vi "TraverseControl_High.vi"(0 "Mode":T1=enum."Read traverse position", 1 "Route Checking?":bool, 3 "Traverse Name":string, 7 "Model       Roll      Pitch       Yaw (deg)":dbl[](array[numeric]) format="%#.2f", 11 "Position input XYZ":dbl[](array[numeric])=[0.0, 0.0, 0.0] format="%.2f", 13 "Speed Factor":dbl=1.0 min=0.1 max=5.0 format="%.2f", 14 "Backlash Compensation?":bool=TRUE) -> (4 "Position Output XYZ":dbl[](array[numeric]) format="%.2f", 15 "Error String":string)   [LabVIEW 2012]
uses:
  Anemometry/Anemometry Sub Vis/Gen Trav/Trav_mode.ctl
  Anemometry/Anemometry Sub Vis/Globals/Trav_pos_global.vi
  Anemometry/Anemometry Sub Vis/Gen Trav/Route mapping/Route_mapping_global.vi
  Anemometry/Anemometry Sub Vis/Globals/Preference_global.vi
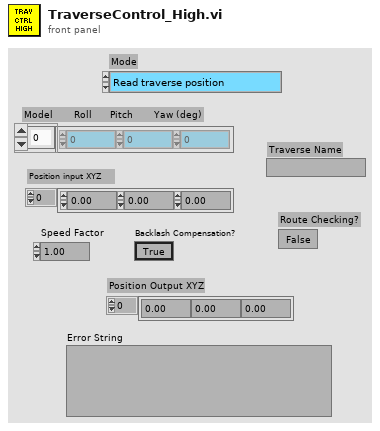
[diagram p1: front panel]
types:
  T1 = typedef "Trav_mode.ctl" = enum16{"Move traverse", "Read traverse position", "Teach Position"}
  T2 = typedef "Tunnel_Coordinates.ctl" = enum16{"Work in Tunnel Coordinates", "Work in Model Coordinates"}
  T3 = typedef "Exclude_cluster.ctl" = cluster{"Sizes":T4, "Name":string, "Exclude Type":T5}
  T4 = typedef "Box_size.ctl" = cluster{"Max":dbl, "Min":dbl}[]
  T5 = typedef "Exclusion_type.ctl" = enum16{"Exclude completely", "Allow only vertical moves"}
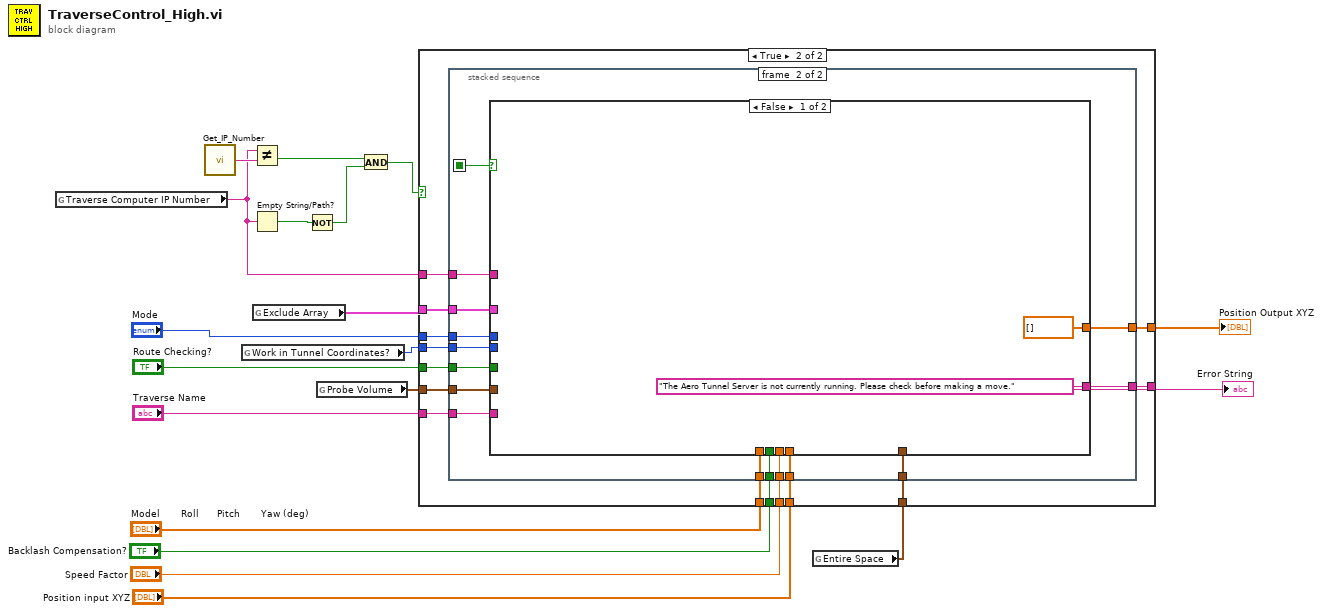
[diagram p0: block diagram]
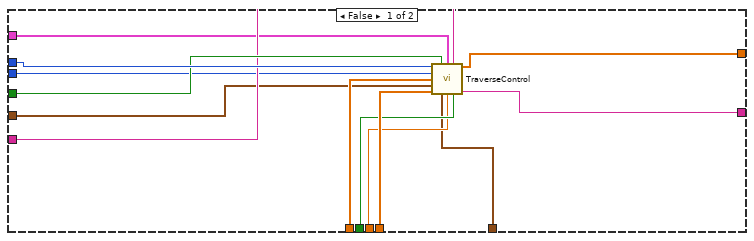
[diagram p2: hidden frame]
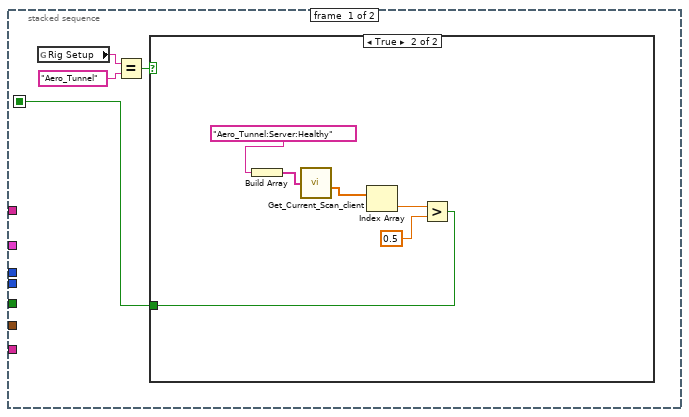
[diagram p3: hidden frame]
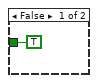
[diagram p4: hidden frame]
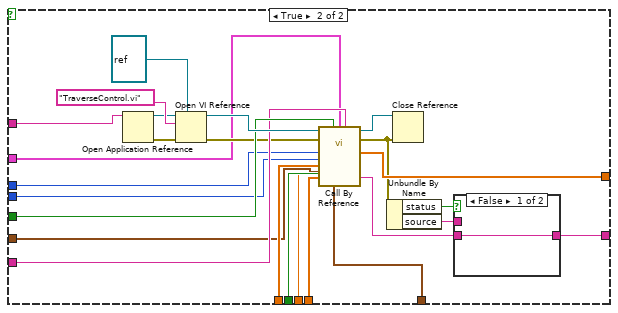
[diagram p5: hidden frame]
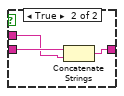
[diagram p6: hidden frame]
diagram:
  n1 = global read "Trav_pos_global.vi" "Traverse Computer IP Number"() -> (w7:string)
  n2 = call "Get_IP_Number.vi"() -> ("IP Number"=w19:string)
  n3 = global read "Trav_pos_global.vi" "Work in Tunnel Coordinates?"() -> (w1:T2)
  n4 = Not Equal?(x=w7, y=w19) -> (x != y?=w6:bool)
  n5 = Empty String/Path?(string/path=w7) -> (empty?=w9:bool)
  n6 = global read "Route_mapping_global.vi" "Exclude Array"() -> (w4:T3[])
  n7 = Not(x=w9) -> (.not. x?=w8:bool)
  n8 = global read "Route_mapping_global.vi" "Probe Volume"() -> (w2:T4)
  n9 = And(x=w6, y=w8) -> (x .and. y?=w5:bool)
  n10 = global read "Route_mapping_global.vi" "Entire Space"() -> (w3:T4)
  n11 = case shown="True" w5 {
    tunnel: "Route Checking?" -> [w25 w46]
    tunnel: "Traverse Name" -> [w24 w45]
    tunnel: [w31 w44] -> w16
    tunnel: [w32 w36] -> w15
    tunnel: "Backlash Compensation?" -> [w28 w43]
    tunnel: "Speed Factor" -> [w27 w42]
    tunnel: "Position input XYZ" -> [w30 w41]
    tunnel: "Model       Roll      Pitch       Yaw (deg)" -> [w29 w40]
    tunnel: "Mode" -> [w26 w39]
    tunnel: w7 -> [_ w38]
    tunnel: w4 -> [w23 w37]
    tunnel: w3 -> [w22 w33]
    tunnel: w2 -> [w21 w34]
    tunnel: w1 -> [w20 w35]
    frame False {
      n12 = call "TraverseControl.vi"("Mode"=w26, "Route Checking?"=w25, "Exclude Array"=w23, "Traverse Name"=w24, "Work in Tunnel Coordinates?"=w20, "Model       Roll      Pitch       Yaw (deg)"=w29, "Probe Volume"=w21, "Position input XYZ"=w30, "Entire Space"=w22, "Speed Factor"=w27, "Backlash Compensation?"=w28) -> ("Position Output XYZ"=w31:dbl[], "Error String"=w32:string)  [unwired: 3 in]
    }
    frame True {
      n13 = stacked-sequence {
        seq-local: [w47 _] -> [_ w58]
        tunnel: w46 -> [_ w72]
        tunnel: w45 -> [_ w71]
        tunnel: [_ w70] -> w44
        tunnel: w43 -> [_ w69]
        tunnel: w42 -> [_ w68]
        tunnel: w41 -> [_ w67]
        tunnel: w40 -> [_ w66]
        tunnel: w39 -> [_ w65]
        tunnel: w38 -> [_ w64]
        tunnel: w37 -> [_ w63]
        tunnel: [_ w62] -> w36
        tunnel: w35 -> [_ w61]
        tunnel: w34 -> [_ w60]
        tunnel: w33 -> [_ w59]
        frame #0 {
          n14 = global read "Preference_global.vi" "Rig Setup"() -> (w50:string)
          n15 = Equal?(x=w50, y="Aero_Tunnel" ("Rig Setup")) -> (x = y?=w48:bool)
          n16 = case shown="True" w48 {
            tunnel: [TRUE w52] -> w47
            frame False {
            }
            frame True {
              n17 = Build Array("Aero_Tunnel:Server:Healthy") -> (w57:string[])
              n18 = call "Get_Current_Scan_client.vi"("ADAM Ch Names"=w57) -> ("Numerical Values"=w55:dbl[])  [unwired: 3 out]
              n19 = Index Array(array=w55) -> (element=w54:dbl)  [unwired: 1 in]
              n20 = Greater?(x=w54, y=0.5) -> (0:w52:bool)
            }
          }
        }
        frame #1 {
          n21 = case shown="False" w58 {
            tunnel: w72 -> [_ w96]
            tunnel: w71 -> [_ w95]
            tunnel: [dbl[] [] ("Position Output XYZ") w94] -> w70
            tunnel: w69 -> [_ w93]
            tunnel: w68 -> [_ w92]
            tunnel: w67 -> [_ w91]
            tunnel: w66 -> [_ w90]
            tunnel: w65 -> [_ w89]
            tunnel: w64 -> [_ w86]
            tunnel: w63 -> [_ w83]
            tunnel: ["The Aero Tunnel Server is not currently running. Please check before making a move." ("Error String") w80] -> w62
            tunnel: w61 -> [_ w77]
            tunnel: w60 -> [_ w76]
            tunnel: w59 -> [_ w75]
            frame False {
            }
            frame True {
              n22 = Open Application Reference(11:w86) -> (0:w84:errorcluster, 3:w85:refnum<vi>)  [unwired: 2 in, 1 out]
              n23 = Open VI Reference(type specifier VI Refnum (for type only)=refnum<vi> refnum ("Scout Server"), application reference (local)=w85, vi path="TraverseControl.vi", error in (no error)=w84) -> (vi reference=w97:refnum<vi>, error out=w88:errorcluster)  [unwired: 2 out]
              n24 = call-by-ref "?"(reference=w97, error in=w88, "Mode"=w89, "Route Checking?"=w96, "Exclude Array"=w83, "Traverse Name"=w95, "Work in Tunnel Coordinates?"=w77, "Model       Roll      Pitch       Yaw (deg)"=w90, "Probe Volume"=w76, "Position input XYZ"=w91, "Entire Space"=w75, "Speed Factor"=w92, "Backlash Compensation?"=w93) -> (reference out=w87:refnum<vi>, error out=w82:errorcluster, "Position Output XYZ"=w94:dbl[], "Error String"=w79:string)  [unwired: 3 in]
              n25 = Unbundle By Name(w82) -> ("status"=w81:bool, "source"=w78:string)
              n26 = Close Reference(reference=w87, error in (no error)=w82) -> ()  [unwired: 1 out]
              n27 = case shown="False" w81 {
                tunnel: [w100 w103] -> w80
                tunnel: w79 -> [w100 w102]
                tunnel: w78 -> [_ w101]
                frame False {
                }
                frame True {
                  n28 = Concatenate Strings(w102, w101) -> (w103:string)
                }
              }
            }
          }
        }
      }
    }
  }
  "Error String" <- w15
  "Position Output XYZ" <- w16
